vi "Write Serialized.vi"(8 "error in (no error)":errorcluster, 10 "Serialized":T1, 11 "FM Sweep in":refnum<class "FM Sweep.lvclass">) -> (0 "error out":errorcluster, 3 "FM Sweep out":refnum<class "FM Sweep.lvclass">)   [LabVIEW 2020, in "FM Sweep.lvclass"]
uses:
  FM Sweep.lvclass
  Serialized.ctl
  FM Sweep.lvclass/FM Sweep.ctl
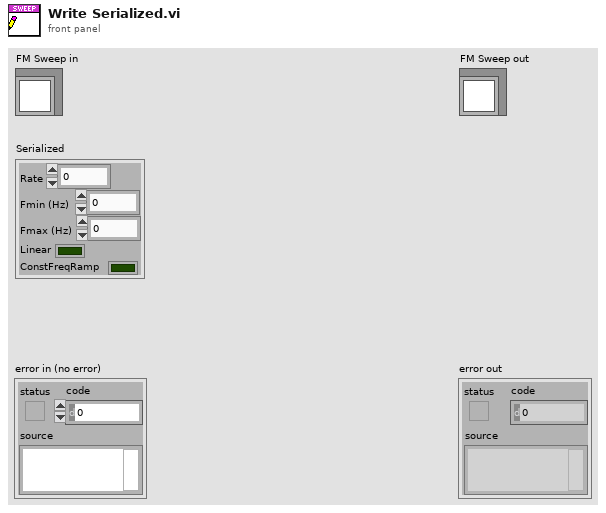
[diagram p1: front panel]
types:
  T1 = typedef "FM Sweep.lvclass/Serialized.ctl" = cluster{"Rate":dbl, "Fmin (Hz)":dbl, "Fmax (Hz)":dbl, "Linear":bool, "ConstFreqRamp":bool}
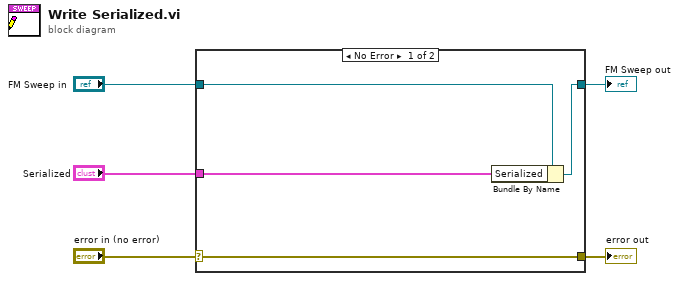
[diagram p0: block diagram]
diagram:
  n1 = case shown="No Error" "error in (no error)" {
    selector: "error in (no error)" -> [w9 w10]
    tunnel: [w9 w10] -> w4
    tunnel: [w7 w11] -> w2
    tunnel: "FM Sweep in" -> [w8 w11]
    tunnel: "Serialized" -> [w6 _]
    frame No Error {
      n2 = Bundle By Name(cluster=w8, "Serialized"=w6) -> (w7:refnum<class "FM Sweep.lvclass">)
    }
    frame Error {
    }
  }
  "error out" <- w4
  "FM Sweep out" <- w2
